vi "SignalGenerator.vi"(10 "Amplitude":dbl, 11 "Frequency":dbl) -> (2 "error out":errorcluster)   [LabVIEW 2014]
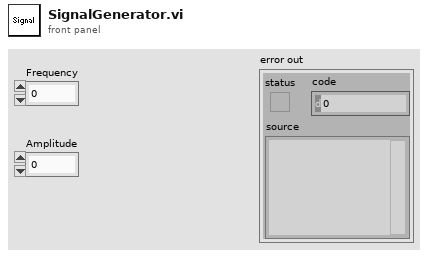
[diagram p1: front panel]
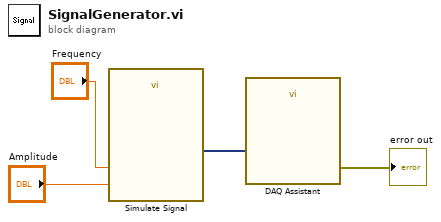
[diagram p0: block diagram]
diagram:
  n1 = call "Simulate Signal"("Frequency"="Frequency", "Amplitude"="Amplitude") -> ("Sine"=w3:dynamicdata)  [unwired: 12 in, 1 out]
  n2 = call "DAQ Assistant"("data"=w3) -> ("error out"=→"error out":errorcluster)  [unwired: 16 in, 2 out]
